vi "cDAQ_VI_Leo_Autotuning.vi"() -> ()   [LabVIEW 2022 SP3]
uses:
  <vilib>/addons/control/pid/autopid.llb/PID autotuning parameters.ctl
  <vilib>/Analysis/baseanly.llb/Mean (DBL).vi
  <vilib>/DAQmx/read.llb/DAQmx Read (Analog 1D Wfm NChan NSamp).vi
  STOP_GLOBAL.vi
  <vilib>/addons/control/pid/pid.llb/PID Lead-Lag (DBL).vi
  <vilib>/addons/control/pid/pid.llb/PID Gain Schedule (DBL).vi
  <vilib>/addons/control/pid/autopid.llb/PID Online Autotuning (Step Closed Loop).vi
  <vilib>/addons/control/pid/pid.llb/PID Advanced (DBL).vi
  <vilib>/addons/control/pid/pid.llb/PID (DBL).vi
  <vilib>/DAQmx/configure/timing.llb/DAQmx Timing (Sample Clock).vi
  <vilib>/DAQmx/miscellaneous.llb/DAQmx Fill In Error Info.vi
  <vilib>/Analysis/NI_AALBase.lvlib
  <vilib>/addons/control/pid/NI_PID_pid.lvlib
  <vilib>/ptbypt/NI_PtbyPt.lvlib
  <vilib>/addons/control/pid/NI_PID_autopid.lvlib
panel:
  in  "MV:":dbl(slide)=30.8641975308642 scale=1.0..5.067 scale format="%.1f"
  in  "autotuning parameters":T1={"type of controller"=0, "relay cycles"=3, "relay amplitude"=1.0, "control specifications"=2, "PV noise level"=0.1} {"PV noise level" format="%.2f"; "control specifications" items=["normal", "fast", "slow"]; "relay amplitude" format="%.2f"; "type of controller" items=["P", "PI", "PID"]}
  in  "PID gain schedule":T2(array[cluster])=[{"PID gains"={"Kc"=7.0, "Ti"=0.001, "Td"=0.0}, "max value"=0.0}] {"max value" format="%.2f"; "PID gains"."Td" format="%#.3g"; "PID gains"."Ti" format="%#.3g"; "PID gains"."Kc" format="%#.3g"}
  out "error out 4":errorcluster
  out "Setpoint profile":dbl
  out "Voltage Output":dynamicdata(graph)
  out "Second Pressure Transducer":cluster{dbl[], dbl[]}(graph)
  out "Second Pressure Transducer":dynamicdata(graph)
  out "Servo Voltage Output":cluster{dbl[], dbl[]}(graph)
  out "Elapsed Time (s)":dbl
  in  "Tab Control":T3(tab)
  in  "Channel Array":dbl[](array[numeric]) format="%_3g"
  out "error out 5":errorcluster
  in  "stop":bool
  out "Output":dbl(slide) scale=1.0..5.067
  out "elapsed time (s)":dbl format="%.3f"
  out "Waveform Chart 2":cluster{"setpoint":dbl, dbl}(graph) caption="Waveform Chart"
  out "Process Variable vs Setpoint":cluster{dbl[], dbl[]}[](graph)
  out "error out":errorcluster
  out "Steps on Needle 3":dbl[](array[numeric])
  in  "Error":dbl
  in  "Scaling Factor":dbl
  in  "x0":dbl
  out "element":dbl
  out "MVT Process variable":dbl
  out "MVT Setpoint":dbl
  out "Gain Index":i32
  in  "SP":dbl format="%.2f"
  out "PID gains out":T4={"proportional gain (Kc)"=1.0, "integral time (Ti, min)"=0.01, "derivative time (Td, min)"=0.0} {"derivative time (Td, min)" format="%.3f"; "integral time (Ti, min)" format="%.3f"; "proportional gain (Kc)" format="%.3f"}
  in  "Insert Gain":bool
  out "output":dbl format="%.2f"
  in  "Autotune":bool
  in  "Reinitialize":bool
  in  "Automatic":bool=TRUE
  in  "Replace Gain":bool
  in  "alpha":dbl=nan format="%.2f"
  out "tuned PID gains":T4={"proportional gain (Kc)"=1.0, "integral time (Ti, min)"=0.01, "derivative time (Td, min)"=0.0} {"derivative time (Td, min)" format="%.3f"; "integral time (Ti, min)" format="%.3f"; "proportional gain (Kc)" format="%.3f"}
  in  "EMERGENCY CLOSE":bool
  out "Steps on Servo":dbl[](array[numeric])
  out "Elapsed Time (s) 2":dbl caption="Elapsed Time (s)"
  out "HAS 3 SECONDS PASSED?":bool
  in  "PRESS TO START":bool
  out "All Channel Graph":cluster{dbl[], dbl[]}[](graph)
  out "Thrust":cluster{dbl[], dbl[]}(graph)
  out "Chamber Pressure":cluster{dbl[], dbl[]}(graph)
  out "Supply Pressure":cluster{dbl[], dbl[]}(graph)
  out "MassFlow":cluster{dbl[], dbl[]}(graph)
  out "Temperature":cluster{dbl[], dbl[]}(graph)
  out "error out 3":errorcluster caption="error out"
  out "error out 2":errorcluster
  in  "rate":dbl=1000.0 format="%0.2f"
  in  "number of samples":i32=100
  in  "File Format":string
  in  "File Name Out":string
  in  "Data Collection Folder":path
  out "Temperature":dynamicdata(graph)
  out "Numeric 2":i32
  out "Thrust lb":dynamicdata(graph)
  in  "Types of Testing":enum32{"Test Firing", "Cold Flow Rig"}(tab)
  out "Saving Data":bool
  out "Filename Out":path
  in  "Collect Data?":bool=TRUE caption="Enable"
  in  "Collect Data? 2":bool=TRUE caption="Enable"
  out "Saving Data":bool
  out "Filename Out":path
  out "Supply Pressure PSI":dynamicdata(graph)
  out "Mass Flow L/min":dynamicdata(graph)
  out "Chamber Pressure":dynamicdata(graph)
  # "Control Loop"
  # "DATA LOGGING INFORMATION"
  # "ANALOG VOLTAGE OUTPUT"
  # "RESULTS"
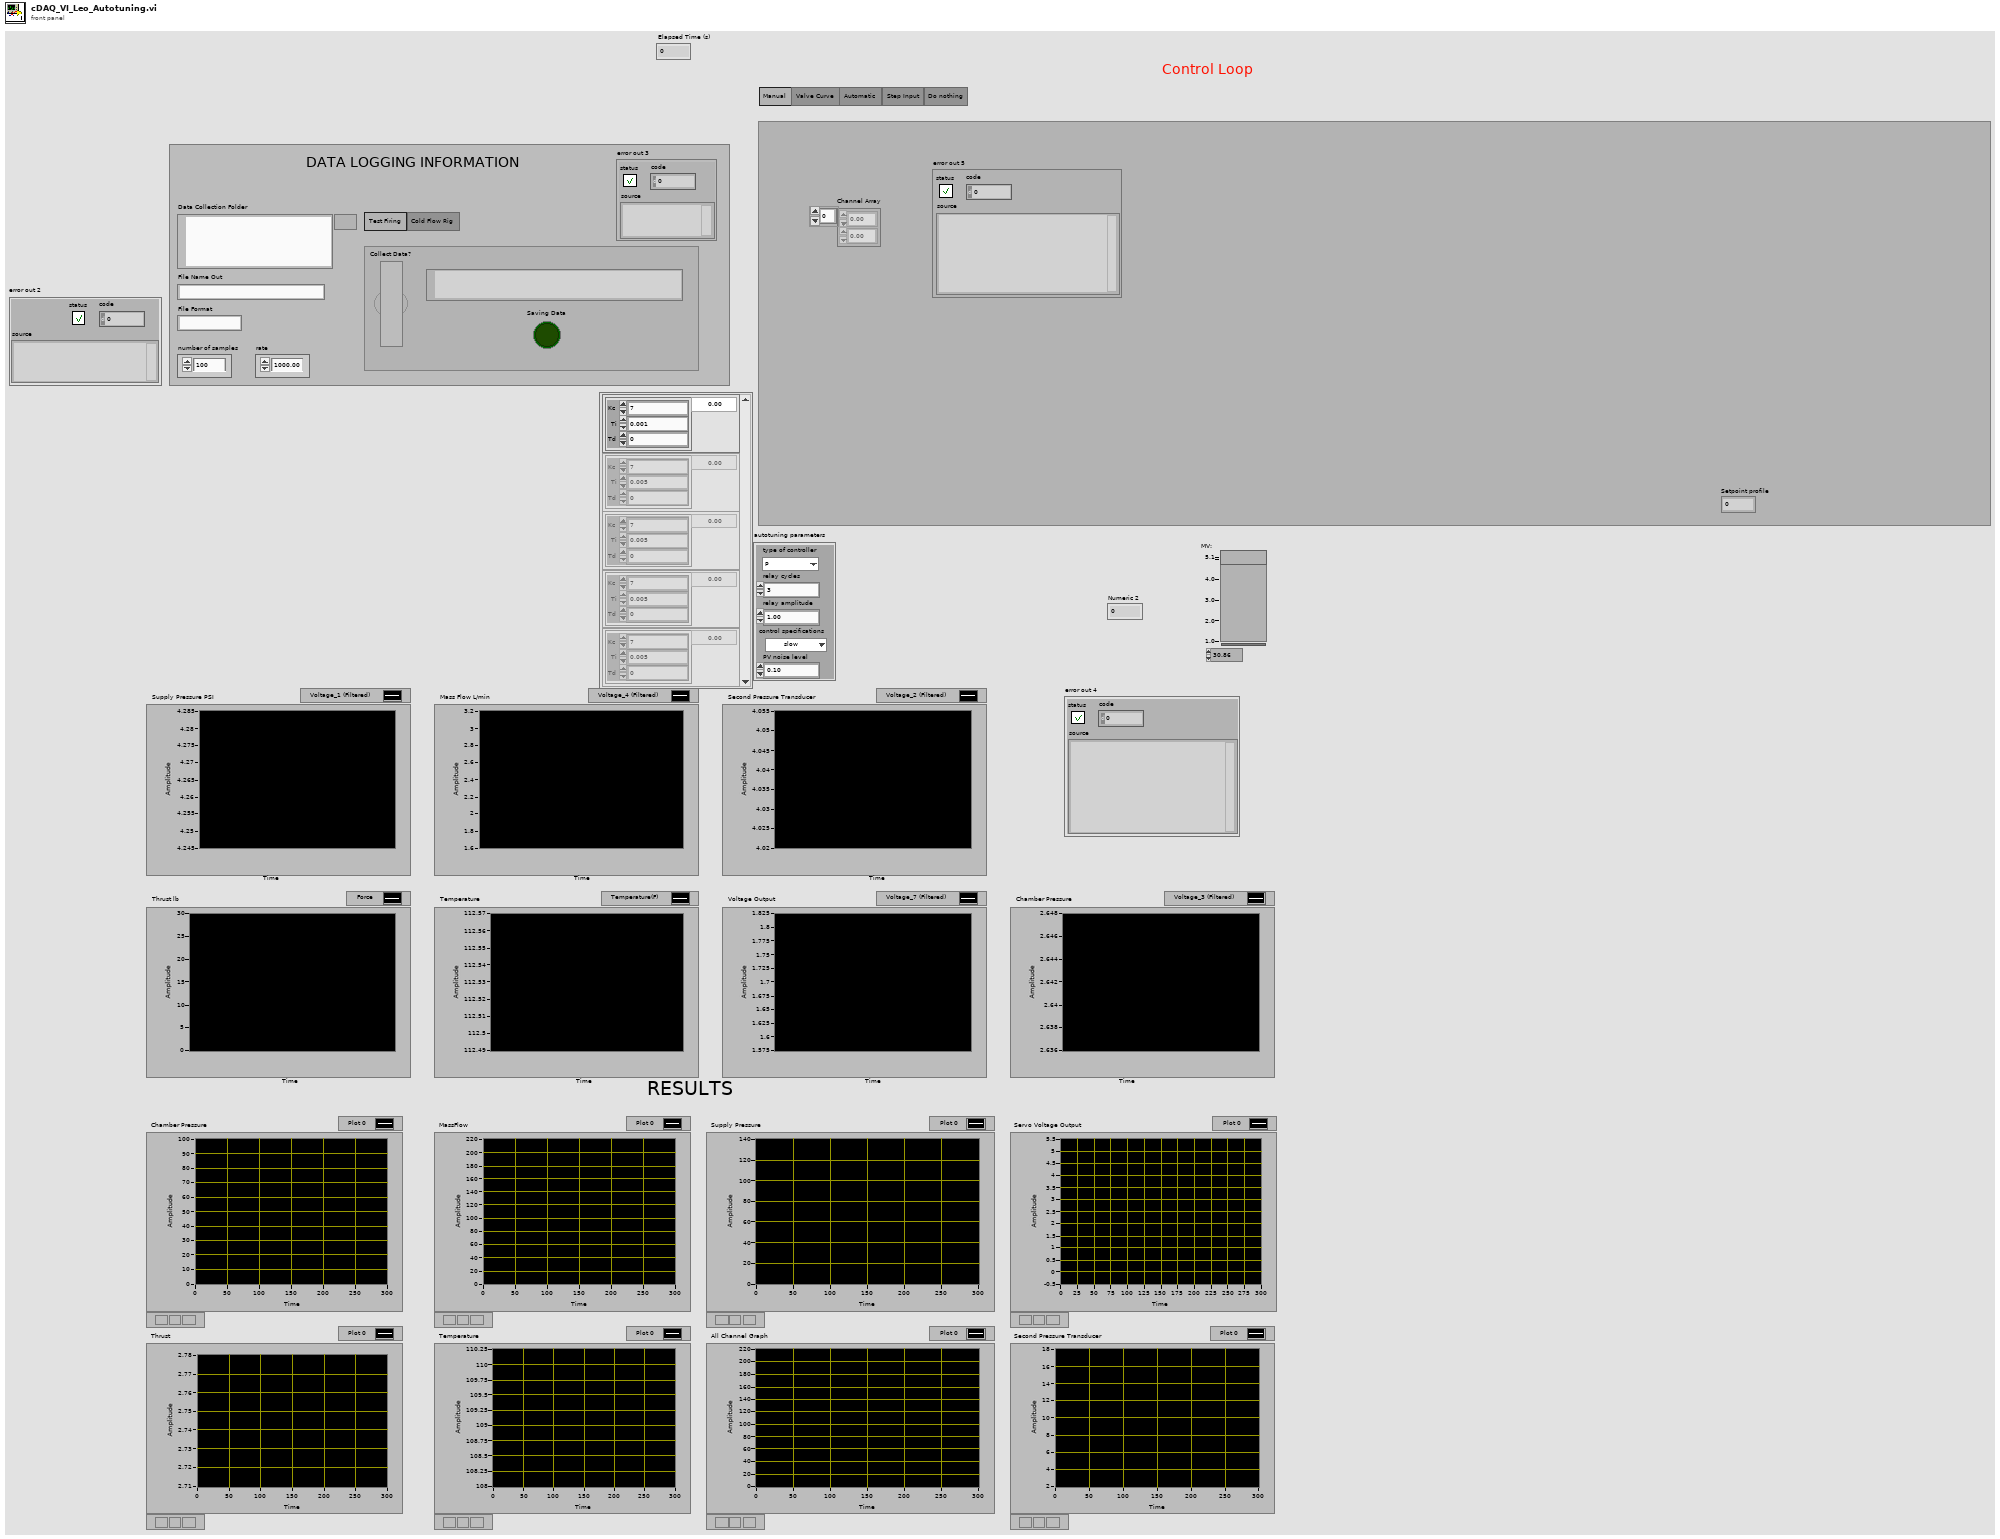
[diagram p1: front panel]
types:
  T1 = typedef "PID autotuning parameters.ctl" = cluster{"type of controller":u16, "relay cycles":i32, "relay amplitude":dbl, "control specifications":u16, "PV noise level":dbl}
  T2 = cluster{"PID gains":cluster{"Kc":dbl, "Ti":dbl, "Td":dbl}, "max value":dbl}[]
  T3 = enum32{"Manual", "Valve Curve", "Automatic", "Step Input", "Do nothing"}
  T4 = cluster{"proportional gain (Kc)":dbl, "integral time (Ti, min)":dbl, "derivative time (Td, min)":dbl}
  T5 = cluster{"tuned PID gains":cluster{"proportional gain (Kc)":dbl, "integral time (Ti, min)":dbl, "derivative time (Td, min)":dbl}, "SP":dbl}
  T6 = cluster{"PID gains":cluster{"Kc":dbl, "Ti":dbl, "Td":dbl}, "max value":dbl}
  T7 = cluster{"tuned PID gains":cluster{"proportional gain (Kc)":dbl, "integral time (Ti, min)":dbl, "derivative time (Td, min)":dbl}, "max value":dbl}
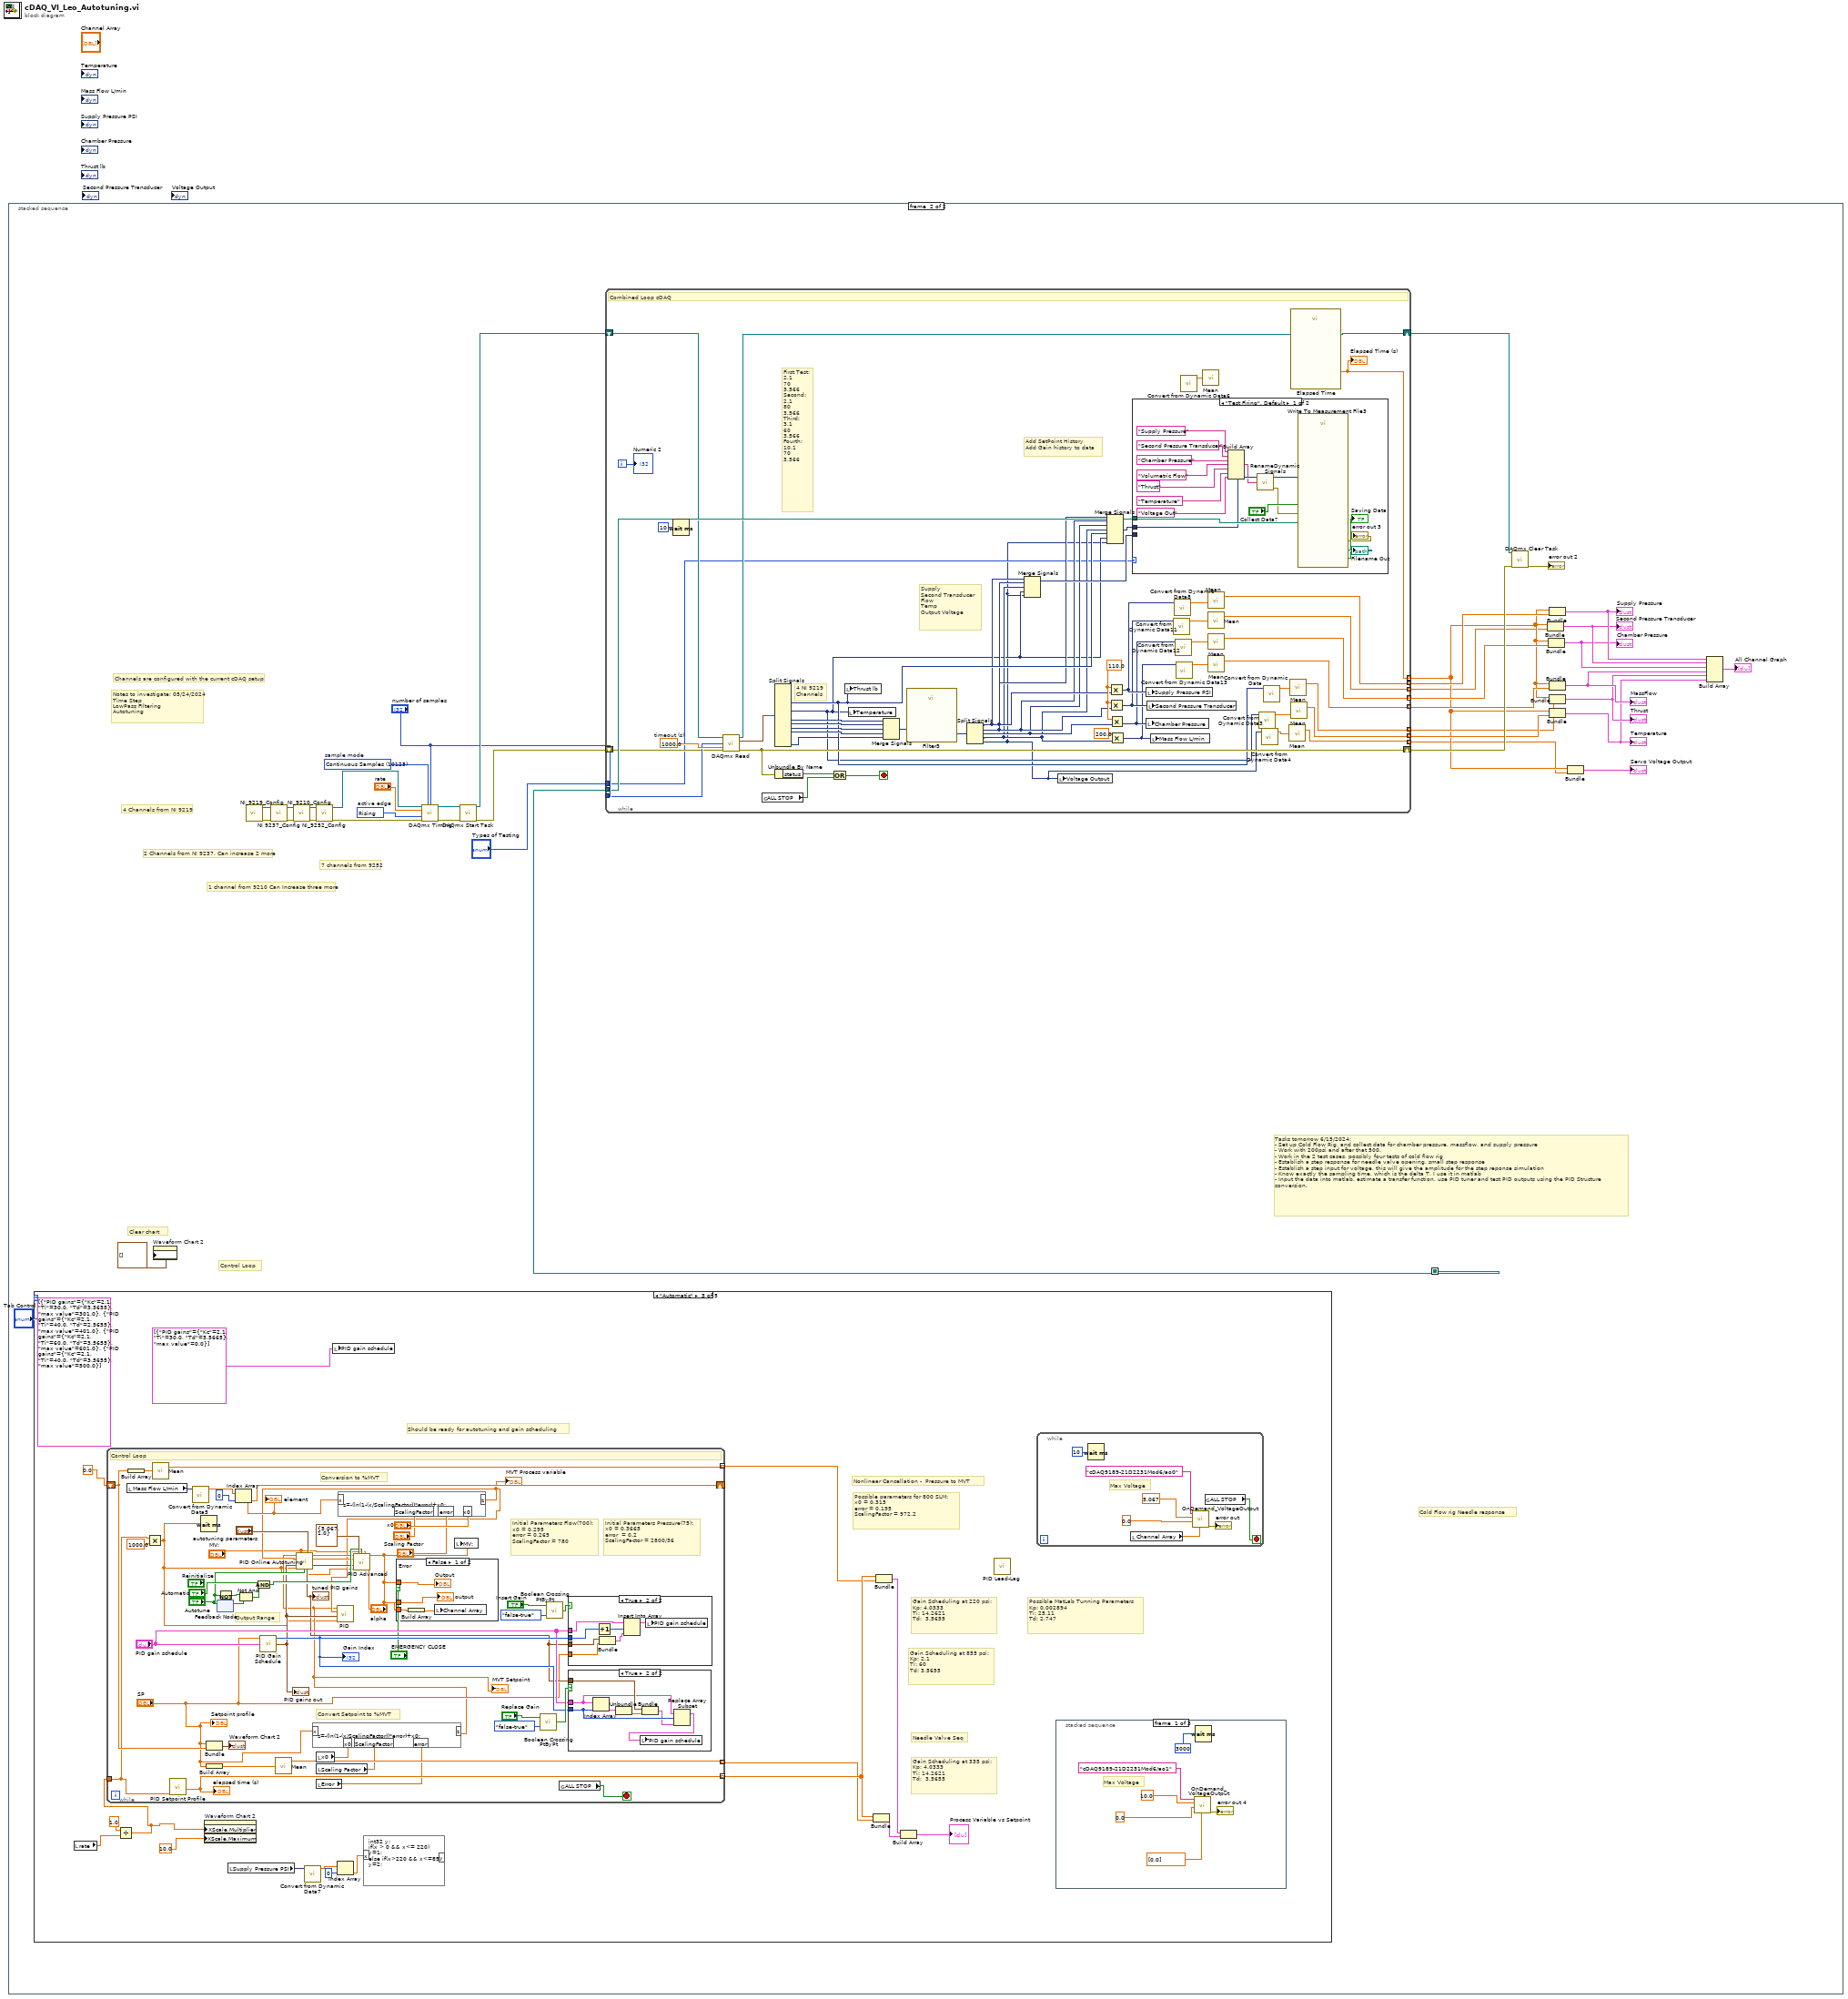
[diagram p0: block diagram]
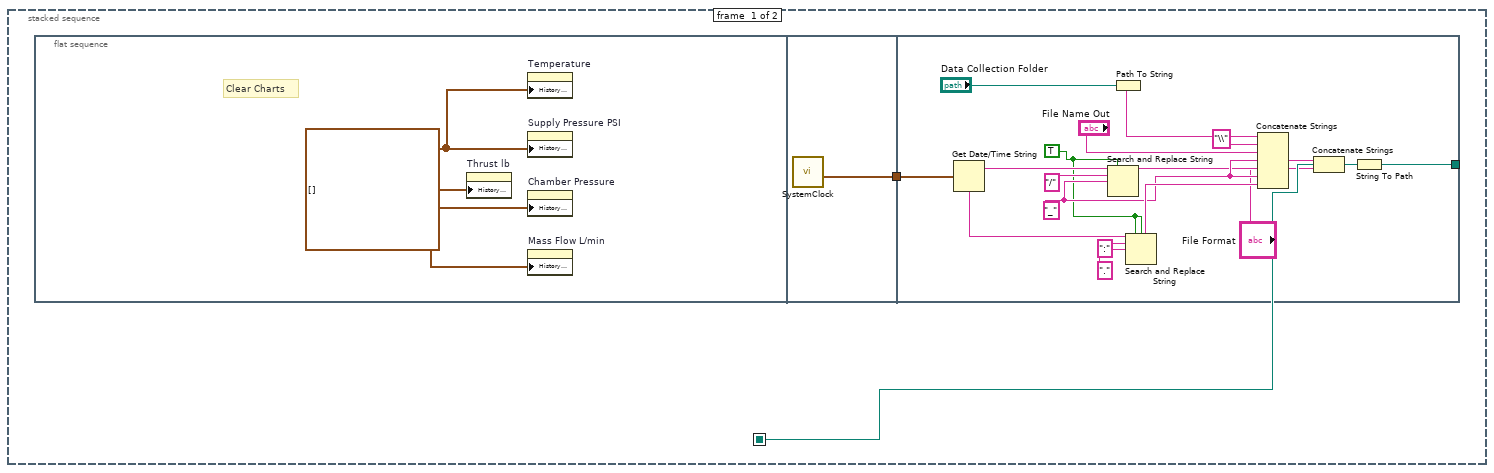
[diagram p2: hidden frame]
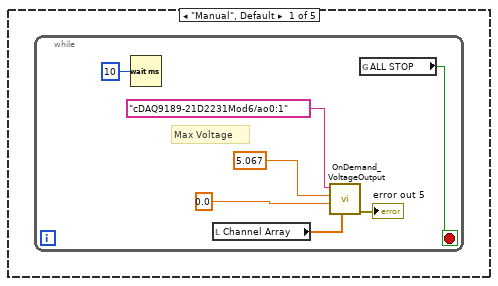
[diagram p3: hidden frame]
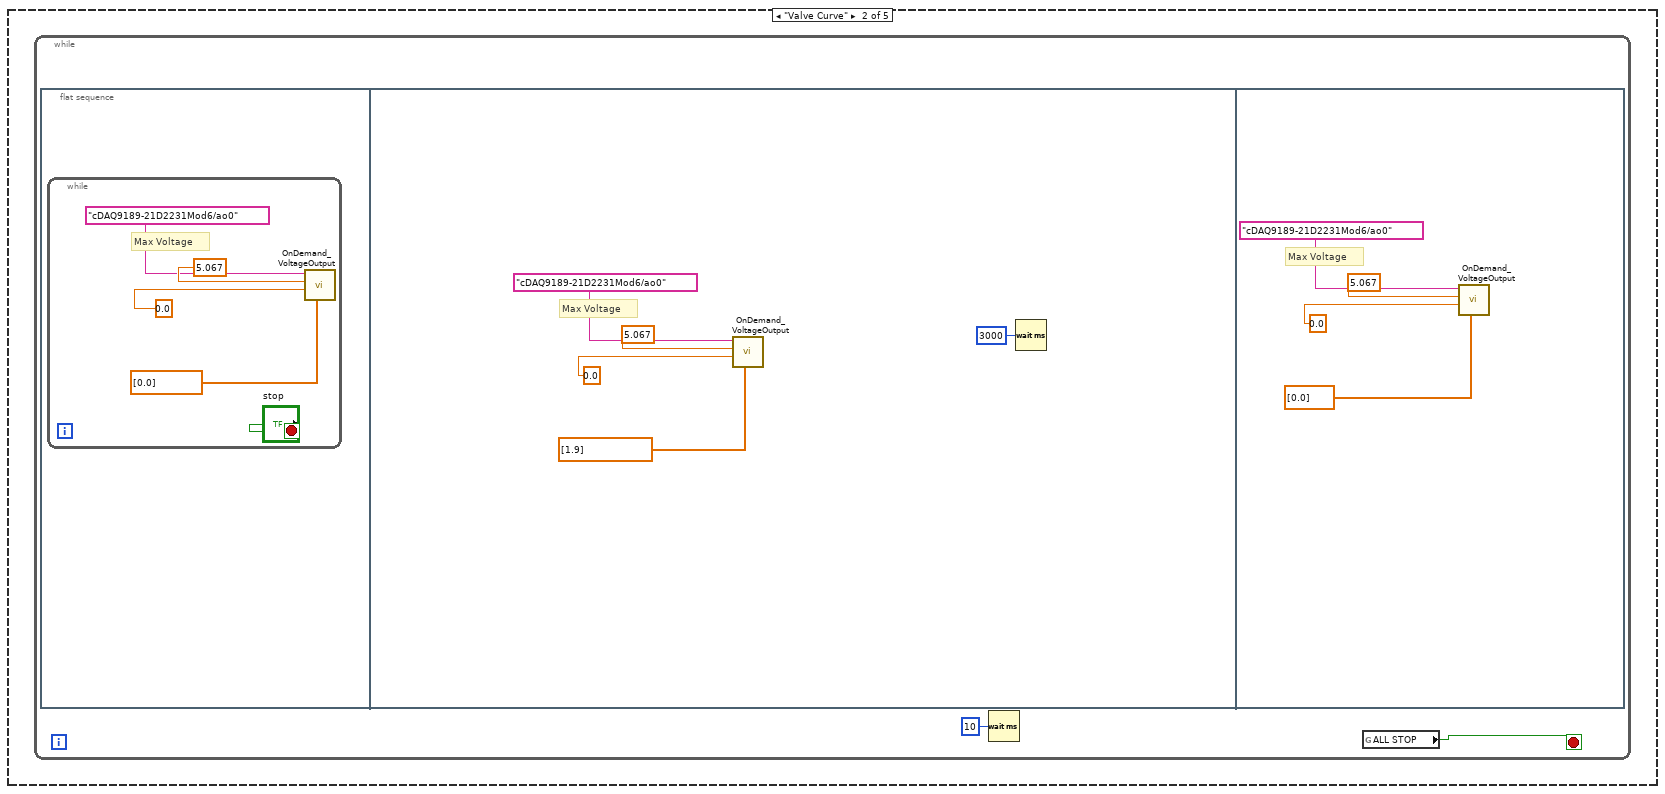
[diagram p4: hidden frame]
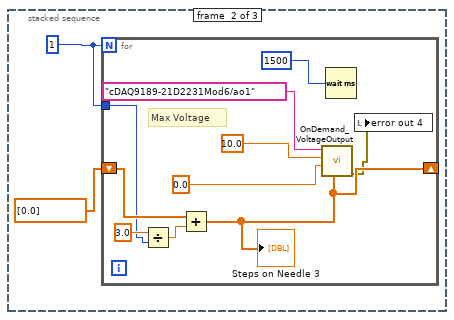
[diagram p5: hidden frame]
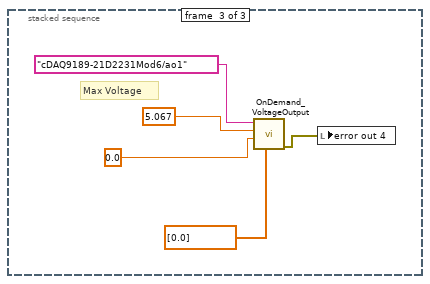
[diagram p6: hidden frame]
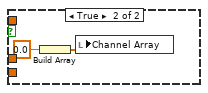
[diagram p7: hidden frame]
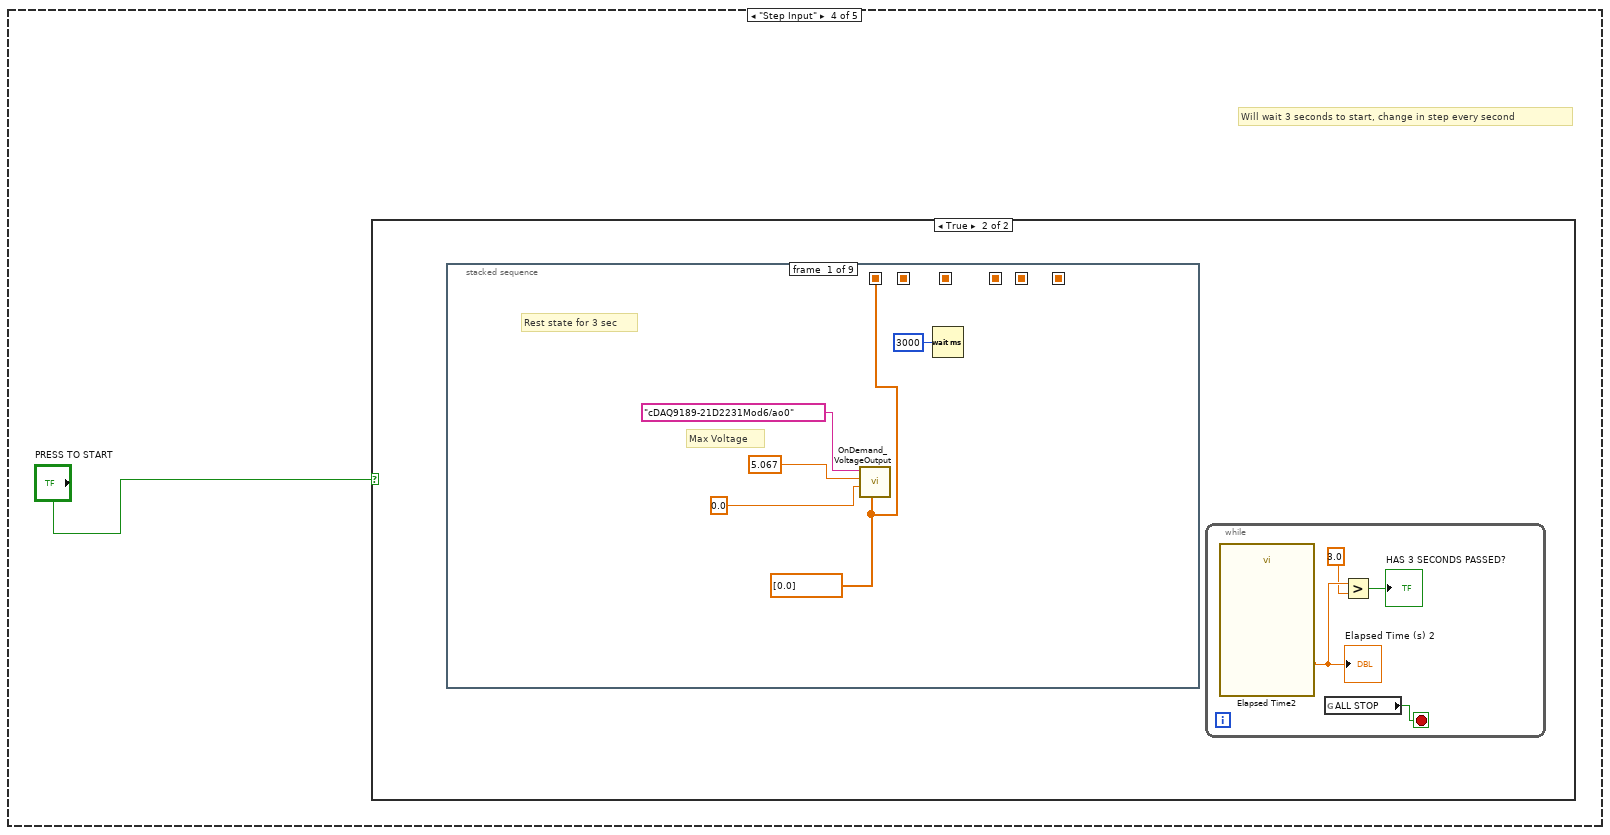
[diagram p10: hidden frame]
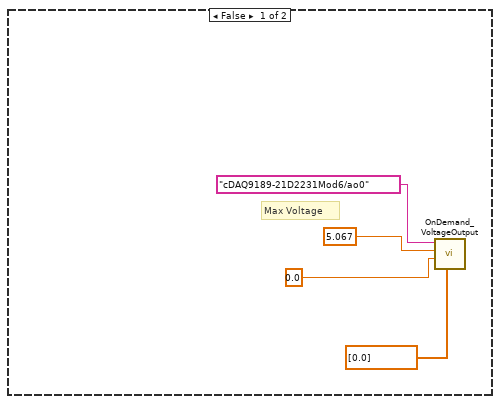
[diagram p11: hidden frame]
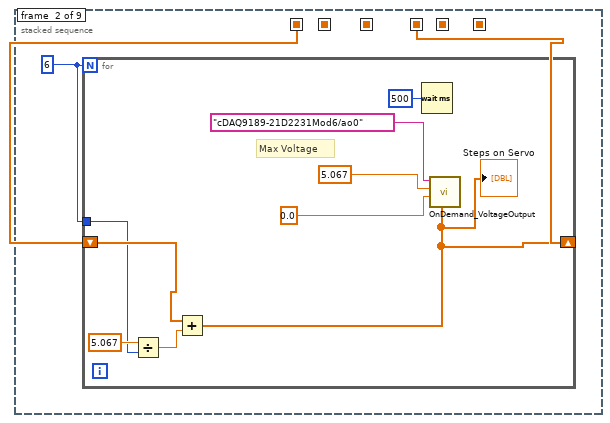
[diagram p12: hidden frame]
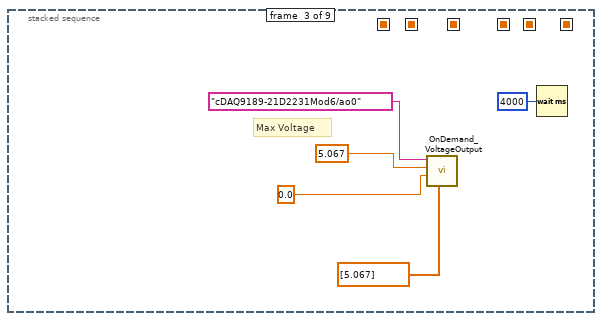
[diagram p13: hidden frame]
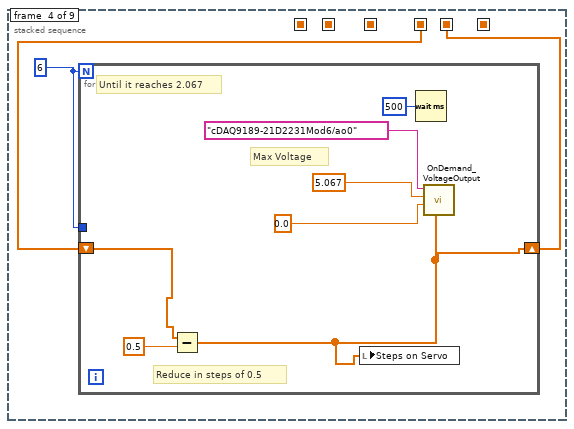
[diagram p14: hidden frame]
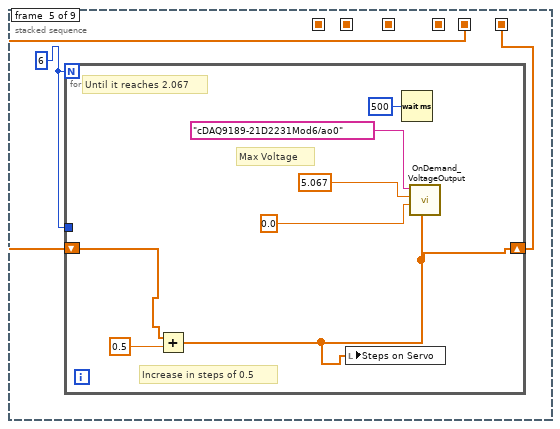
[diagram p15: hidden frame]
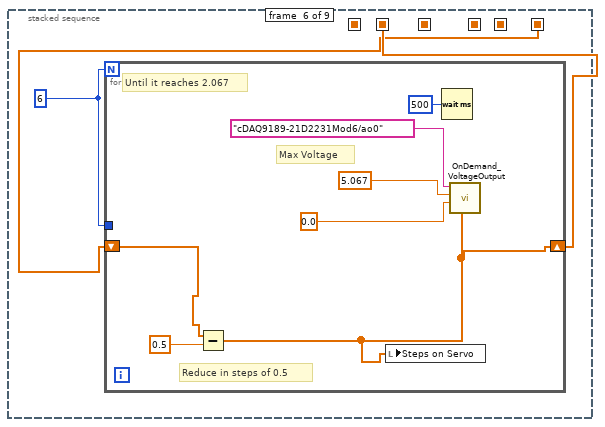
[diagram p16: hidden frame]
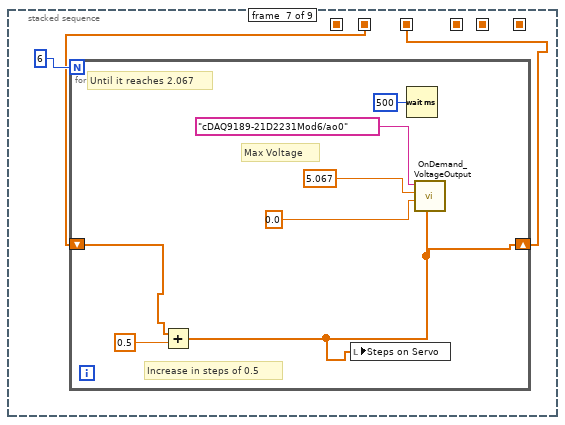
[diagram p17: hidden frame]
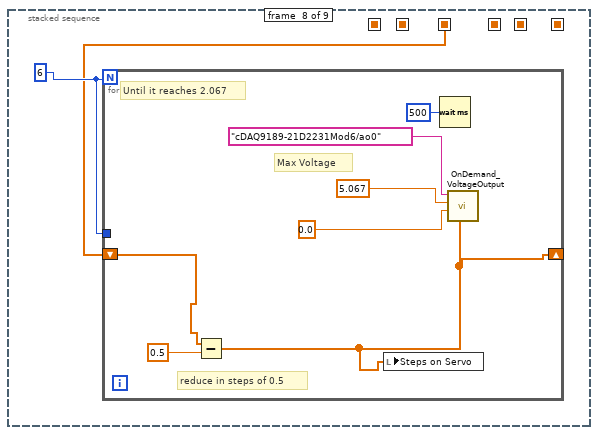
[diagram p18: hidden frame]
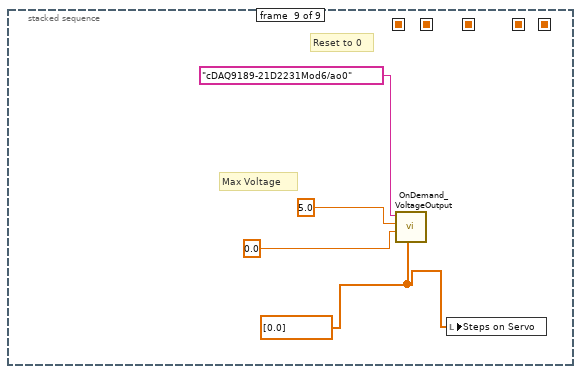
[diagram p19: hidden frame]
diagram:
  n1 = stacked-sequence {
    seq-local: [w1 _] -> [_ w60]
    frame #0 {
      n2 = flat-sequence {
        tunnel: [w4] -> w2
        tunnel: w2 -> [w11]
        tunnel: [w10] -> w1
        frame #0 {
          w3 = waveform(dbl)[] []
          # "Clear Charts"
          n3 = property on="Thrust lb" class="WFChart (strict)"("History Data"=w3) -> ()  [unwired: 2 in, 2 out]
          n4 = property on="Temperature" class="WFChart (strict)"("History Data"=w3) -> ()  [unwired: 2 in, 2 out]
          n5 = property on="Supply Pressure PSI" class="WFChart (strict)"("History Data"=w3) -> ()  [unwired: 2 in, 2 out]
          n6 = property on="Chamber Pressure" class="WFChart (strict)"("History Data"=w3) -> ()  [unwired: 2 in, 2 out]
          n7 = property on="Mass Flow L/min" class="WFChart (strict)"("History Data"=w3) -> ()  [unwired: 2 in, 2 out]
        }
        frame #1 {
          n8 = call "SystemClock.vi"() -> ("LabVIEW Time Stamp"=w4:timestamp)  [unwired: 9 in, 2 out]
        }
        frame #2 {
          w6 = TRUE ("replace all? (F)")
          w19 = "_" ("string")
          n9 = Get Date/Time String(seconds (now)=w11) -> (date string=w13:string, time string=w16:string)  [unwired: 2 in]
          n10 = Search and Replace String(replace all?=w6, input string=w13, search string="/", replace string=w19) -> (result string=w15:string)  [unwired: 4 in, 3 out]
          n11 = Path To String(path="Data Collection Folder") -> (string=w8:string)
          n12 = Search and Replace String(replace all?=w6, case sensitive?=w6, input string=w16, search string=":", replace string="." ("replace string (\"\")")) -> (result string=w20:string)  [unwired: 3 in, 3 out]
          n13 = Concatenate Strings(w8, "\\" ("string"), "File Name Out", w19, w15, w19, w20) -> (w21:string)
          n14 = Concatenate Strings(w21, "File Format") -> (w22:string)
          n15 = String To Path(string=w22) -> (path=w10:path)
        }
      }
    }
    frame #1 {
      w58 = 10123 items=["Finite Samples"=10178, "Continuous Samples"=10123, "Hardware Timed Single Point"=12522]  # sample mode
      w59 = 10280 items=["Rising"=10280, "Falling"=10171]  # active edge
      # "Cold Flow rig Needle response"
      # "Tasks tomorrow 6/15/2024:\n- Set up Cold Flow Rig, and collect data for chamber pressure, massflow, and supply pressure\n- Work with 200psi and after that 500.\n- Work in the 2 test cases, possibly four tests of cold flow rig\n- Establish a step response for needle valve opening, small step response\n- Establish a step input for voltage, this will give the amplitude for the step reponse simulation\n- Know exactly the sampling time, which is the delta T, I use it in matlab\n- Input the data into matlab, estimate a transfer function, use PID tuner and test PID outputs using the PID Structure\nconversion."
      # "Control Loop"
      # "Clear chart"
      # "Notes to investigate: 05/24/2024\nTime Step\nLowPass FIltering\nAutotuning"
      # "Channels are configured with the current cDAQ setup"
      # "7 channels from 9252"
      # "1 channel from 9210 Can Increase three more"
      # "2 Channels from NI 9237, Can increase 2 more"
      # "4 Channels from NI 9219"
      n16 = case shown="\"Automatic\"" "Tab Control" {
        frame "Manual", Default {
          n17 = while {
            stop <- w68 stop-if-true
            # "Max Voltage"
            n18 = Wait (ms)(milliseconds to wait=u32 10) -> ()  [unwired: 1 out]
            n19 = local read "Channel Array"() -> (w64:dbl[])
            n20 = call "OnDemand_VoltageOutput.vi"("Channel Array"=w64, "minimum voltage"=0.0, "maximum voltage"=5.067, "physical channels"="cDAQ9189-21D2231Mod6/ao0:1") -> ("error out"=→"error out 5":errorcluster)  [unwired: 7 in]
            n21 = global read "STOP_GLOBAL.vi" "ALL STOP"() -> (w68:bool)
          }
        }
        frame "Valve Curve" {
          n22 = while {
            stop <- w69 stop-if-true
            n23 = flat-sequence {
              frame #0 {
                n24 = while {
                  stop <- "stop" stop-if-true
                  # "Max Voltage"
                  n25 = call "OnDemand_VoltageOutput.vi"("Channel Array"=dbl[] [0.0], "minimum voltage"=0.0, "maximum voltage"=5.067, "physical channels"="cDAQ9189-21D2231Mod6/ao0") -> ()  [unwired: 7 in, 1 out]
                }
              }
              frame #1 {
                # "Max Voltage"
                n26 = call "OnDemand_VoltageOutput.vi"("Channel Array"=dbl[] [1.9], "minimum voltage"=0.0, "maximum voltage"=5.067, "physical channels"="cDAQ9189-21D2231Mod6/ao0") -> ()  [unwired: 7 in, 1 out]
                n27 = Wait (ms)(milliseconds to wait=u32 3000) -> ()  [unwired: 1 out]
              }
              frame #2 {
                # "Max Voltage"
                n28 = call "OnDemand_VoltageOutput.vi"("Channel Array"=dbl[] [0.0], "minimum voltage"=0.0, "maximum voltage"=5.067, "physical channels"="cDAQ9189-21D2231Mod6/ao0") -> ()  [unwired: 7 in, 1 out]
              }
            }
            n29 = Wait (ms)(milliseconds to wait=u32 10) -> ()  [unwired: 1 out]
            n30 = global read "STOP_GLOBAL.vi" "ALL STOP"() -> (w69:bool)
          }
        }
        frame "Automatic" {
          (unwired) T2 [{"PID gains"={"Kc"=2.1, "Ti"=30.0, "Td"=3.5655}, "max value"=301.0}, {"PID gains"={"Kc"=2.1, "Ti"=40.0, "Td"=2.5655}, "max value"=401.0}, {"PID gains"={"Kc"=2.1, "Ti"=60.0, "Td"=3.5655}, "max value"=601.0}, {"PID gains"={"Kc"=2.1, "Ti"=40.0, "Td"=3.5655}, "max value"=500.0}] ("PID gain schedule 2")
          # "Should be ready for autotuning and gain scheduling"
          # "Possible parameters for 800 SLM:\nx0 = 0.315\nerror = 0.195\nScalingFactor = 972.2"
          # "Nonlinear Cancellation -  Pressure to MVT"
          # "Possible MatLab Tunning Parameters\nKp: 0.002894\nTi: 25.11\nTd: 2.747"
          # "Gain Scheduling at 335 psi:\nKp: 4.0333\nTi: 14.2621\nTd:  3.5655"
          # "Gain Scheduling at 855 psi:\nKp: 2.1\nTi: 60\nTd: 3.5655"
          # "Gain Scheduling at 220 psi:\nKp: 4.0333\nTi: 14.2621\nTd:  3.5655"
          # "Needle Valve Seq"
          n31 = local read "rate"() -> (w85:dbl)
          n32 = Divide(x=1.0, y=w85) -> (x/y=w88:dbl)
          n33 = while {
            shift-right: [w138] -> _
            shift-left: 0.0 -> [w176]
            tunnel: w88 -> [w139]
            tunnel: [w177] -> w97 mode=indexing
            tunnel: [w175] -> w95 mode=indexing
            tunnel: [w173] -> w96 mode=indexing
            stop <- w179 stop-if-true
            # "Initial Parameters Pressure(75):\nx0 = 0.3665\nerror  = 0.2\nScalingFactor = 2800/36"
            # "Initial Parameters Flow(700):\nx0 = 0.295\nerror = 0.265\nScalingFactor = 780"
            # "Convert Setpoint to %MVT"
            # "Conversion to %MVT"
            # "Output Range"
            # "Control Loop"
            n34 = local read "Mass Flow L/min"() -> (w163:dynamicdata)
            n35 = Build Array(w176) -> (w174:dbl[])
            n36 = Multiply(x=w139, y=1000.0) -> (x*y=w131:dbl)
            n37 = call-poly <vilib>:"Mean.vi"("X"=w174) -> ("mean"=w175:dbl)  [unwired: 1 out]
            n38 = call <vilib>:"PID Setpoint Profile.vi"("dt (s)"=w139) -> ("elapsed time (s)"=w177:dbl)  [unwired: 5 in, 3 out]
            "elapsed time (s)" <- w177
            n39 = call "Convert from Dynamic Data5"("Dynamic Data Type"=w163) -> ("Array"=w164:dbl[])  [unwired: 3 in]
            n40 = Wait (ms)(milliseconds to wait=w131) -> ()  [unwired: 1 out]
            n41 = Bundle("SP"="SP", w176) -> (→"Waveform Chart 2":cluster{"SP":dbl, dbl})  [unwired: 1 in]
            n42 = Build Array("SP") -> (w170:dbl[])
            n43 = feedback #1() -> (w158:bool)  [unwired: 1 in]
            n44 = feedback-in #1("Autotune") -> ()
            n45 = Not(x="Autotune") -> (.not. x?=w157:bool)
            n46 = Index Array(array=w164, index=0) -> (element=w138:dbl)
            "element" <- w138
            n47 = Not And(1:w158, 2:w157) -> (0:w156:bool)
            n48 = And(x="Automatic", y=w156) -> (x .and. y?=w152:bool)
            n49 = call-poly <vilib>:"PID Gain Schedule.vi"("PID gain schedule"="PID gain schedule", "gain scheduling value"="SP") -> ("PID gains out"=w142:T4, "index out"=w144:i32)  [unwired: 2 in]
            "Gain Index" <- w144
            "PID gains out" <- w142
            n50 = call-poly <vilib>:"Mean.vi"("X"=w170) -> ("mean"=w173:dbl)  [unwired: 1 out]
            n51 = local read "x0"() -> (w169:dbl)
            n52 = local read "Scaling Factor"() -> (w159:dbl)
            n53 = local read "Error"() -> (w168:dbl)
            n54 = formula code="z=-(ln(1-(x/ScalingFactor))*error)+x0;"("x"="SP", "x0"=w169, "ScalingFactor"=w159, "error"=w168) -> ("z"=w135:dbl)
            "MVT Setpoint" <- w135
            n55 = formula code="z=-(ln(1-(x/ScalingFactor))*error)+x0;"("x"=w138, "x0"="x0", "ScalingFactor"="Scaling Factor", "error"="Error") -> ("z"=w137:dbl)
            "MVT Process variable" <- w137
            n56 = call-poly <vilib>:"PID Online Autotuning.vi"("setpoint"=w135, "manipulated variable"="MV:", "autotuning parameters"="autotuning parameters", "process variable"=w137, "PID gains in"=w142, "dt (s)"=w131, "autotune? (F)"="Autotune") -> ("setpoint out"=w151:dbl, "process variable out"=w150:dbl, "PID gains out"=w149:T4, "tuned PID gains"=w140:T4)  [unwired: 4 in, 1 out]
            "tuned PID gains" <- w140
            n57 = call-poly <vilib>:"PID.vi"("dt (s)"=w131, "PID gains"=w142, "process variable"=w137, "setpoint"=w135) -> ()  [unwired: 6 in, 2 out]
            n58 = call-poly <vilib>:"PID Advanced.vi"("setpoint"=w151, "output range"=cluster{"output high":dbl, "output low":dbl} {"output high"=5.067, "output low"=1.0}, "auto? (T)"=w152, "manual control"="MV:", "process variable"=w150, "alpha"="alpha", "PID gains"=w149, "dt (s)"=w131) -> ("output"=w132:dbl)  [unwired: 6 in, 1 out]
            n59 = case shown="False" "EMERGENCY CLOSE" {
              tunnel: w132 -> [w183 _]
              tunnel: w132 -> [w182 _]
              tunnel: w132 -> [w180 _]
              frame False {
                n60 = Build Array(w180) -> (w181:dbl[])
                n61 = local write "Channel Array"(w181) -> ()
                "Output" <- w183
                "output" <- w182
              }
              frame True {
                n62 = Build Array(0.0 ("element")) -> (w185:dbl[])
                n63 = local write "Channel Array"(w185) -> ()
              }
            }
            n64 = local write "MV:"(w132) -> ()
            n65 = call <vilib>:"Boolean Crossing PtByPt.vi"("direction"=enum16{"either", "false-true", "true-false"}."false-true", "input"="Replace Gain") -> ("crossing"=w145:bool)  [unwired: 1 in]
            n66 = call <vilib>:"Boolean Crossing PtByPt.vi"("direction"=enum16{"either", "false-true", "true-false"}."false-true", "input"="Insert Gain") -> ("crossing"=w161:bool)  [unwired: 1 in]
            n67 = global read "STOP_GLOBAL.vi" "ALL STOP"() -> (w179:bool)
            n68 = case shown="True" w161 {
              tunnel: w144 -> [_ w199]
              tunnel: "PID gain schedule" -> [_ w197]
              tunnel: "SP" -> [_ w196]
              tunnel: w140 -> [_ w194]
              frame False {
              }
              frame True {
                n69 = Increment(x=w199) -> (x+1=w198:i32)
                n70 = Bundle("tuned PID gains"=w194, "SP"=w196) -> (w193:T5)  [unwired: 1 in]
                n71 = Insert Into Array(array=w197, index=w198, new element=w193) -> (w195:T2)
                n72 = local write "PID gain schedule"(w195) -> ()
              }
            }
            n73 = case shown="True" w145 {
              tunnel: w144 -> [_ w189]
              tunnel: "PID gain schedule" -> [_ w187]
              tunnel: w140 -> [_ w190]
              frame False {
              }
              frame True {
                n74 = Index Array(array=w187, index=w189) -> (element=w192:T6)
                n75 = Unbundle(w192) -> ("max value"=w191:dbl)  [unwired: 1 out]
                n76 = Bundle("tuned PID gains"=w190, "max value"=w191) -> (w188:T7)  [unwired: 1 in]
                n77 = Replace Array Subset(array=w187, new element=w188, index=w189) -> (w186:T2)
                n78 = local write "PID gain schedule"(w186) -> ()
              }
            }
            "Setpoint profile" <- "SP"
          }
          n79 = property on="Waveform Chart 2" class="WFChart (strict)"("XScale.Multiplier"=w88, "XScale.Maximum"=10.0 ("X Scale.Range:Maximum")) -> ()  [unwired: 2 in, 2 out]
          n80 = local read "Supply Pressure PSI"() -> (w92:dynamicdata)
          n81 = call "Convert from Dynamic Data7"("Dynamic Data Type"=w92) -> ("Array"=w91:dbl[])  [unwired: 3 in]
          n82 = local write "PID gain schedule"(T2 [{"PID gains"={"Kc"=2.1, "Ti"=30.0, "Td"=3.5665}, "max value"=0.0}] ("PID gain schedule 2")) -> ()
          n83 = Index Array(array=w91, index=0) -> (element=w89:dbl)
          n84 = formula code="int32 y;\nif(x > 0 && x<= 220)\ny=1;\nelse if(x>220 && x<=855)\ny=2;"("x"=w89) -> ()  [unwired: 1 out]
          n85 = Bundle(w97, w96) -> (w98:cluster{dbl[], dbl[]})  [unwired: 1 in]
          n86 = Bundle(w97, w95) -> (w93:cluster{dbl[], dbl[]})  [unwired: 1 in]
          n87 = Build Array(w93, w98) -> (→"Process Variable vs Setpoint":cluster{dbl[], dbl[]}[])
          n88 = call-poly <vilib>:"PID Lead-Lag.vi"() -> ()  [unwired: 8 in, 2 out]
          n89 = while {
            stop <- w130 stop-if-true
            # "Max Voltage"
            n90 = Wait (ms)(milliseconds to wait=u32 10) -> ()  [unwired: 1 out]
            n91 = local read "Channel Array"() -> (w126:dbl[])
            n92 = call "OnDemand_VoltageOutput.vi"("Channel Array"=w126, "minimum voltage"=0.0, "maximum voltage"=5.067, "physical channels"="cDAQ9189-21D2231Mod6/ao0") -> ("error out"=→"error out":errorcluster)  [unwired: 7 in]
            n93 = global read "STOP_GLOBAL.vi" "ALL STOP"() -> (w130:bool)
          }
          n94 = stacked-sequence {
            frame #0 {
              # "Max Voltage"
              n95 = call "OnDemand_VoltageOutput.vi"("Channel Array"=dbl[] [0.0], "minimum voltage"=0.0, "maximum voltage"=10.0, "physical channels"="cDAQ9189-21D2231Mod6/ao1") -> ("error out"=→"error out 4":errorcluster)  [unwired: 7 in]
              n96 = Wait (ms)(milliseconds to wait=u32 3000) -> ()  [unwired: 1 out]
            }
            frame #1 {
              w107 = 1
              n97 = for {
                N: w107 -> [_]
                shift-right: [w110] -> _
                shift-left: dbl[] [0.0] -> [w114]
                tunnel: w107 -> [w112]
                # "Max Voltage"
                n98 = Divide(x=3.0, y=w112) -> (x/y=w111:dbl)
                n99 = Add(x=w114, y=w111) -> (x+y=w110:dbl[])
                "Steps on Needle 3" <- w110
                n100 = call "OnDemand_VoltageOutput.vi"("Channel Array"=w110, "minimum voltage"=0.0, "maximum voltage"=10.0, "physical channels"="cDAQ9189-21D2231Mod6/ao1") -> ("error out"=w109:errorcluster)  [unwired: 7 in]
                n101 = Wait (ms)(milliseconds to wait=u32 1500) -> ()  [unwired: 1 out]
                n102 = local write "error out 4"(w109) -> ()
              }
            }
            frame #2 {
              # "Max Voltage"
              n103 = call "OnDemand_VoltageOutput.vi"("Channel Array"=dbl[] [0.0], "minimum voltage"=0.0, "maximum voltage"=5.067, "physical channels"="cDAQ9189-21D2231Mod6/ao1") -> ("error out"=w119:errorcluster)  [unwired: 7 in]
              n104 = local write "error out 4"(w119) -> ()
            }
          }
        }
        frame "Step Input" {
          # "Will wait 3 seconds to start, change in step every second"
          n105 = case shown="True" "PRESS TO START" {
            frame False {
              # "Max Voltage"
              n106 = call "OnDemand_VoltageOutput.vi"("Channel Array"=dbl[] [0.0], "minimum voltage"=0.0, "maximum voltage"=5.067, "physical channels"="cDAQ9189-21D2231Mod6/ao0") -> ()  [unwired: 7 in, 1 out]
            }
            frame True {
              n107 = stacked-sequence {
                seq-local: [_ _ _ _ _ w252 _ _ _] -> [_ _ _ _ _ _ w262 _ _]
                seq-local: [_ _ _ _ _ _ w261 _ _] -> [_ _ _ _ _ _ _ w271 _]
                seq-local: [w209 _ _ _ _ _ _ _ _] -> [_ w215 _ _ _ _ _ _ _]
                seq-local: [_ w214 _ _ _ _ _ _ _] -> [_ _ _ w232 _ _ _ _ _]
                seq-local: [_ _ _ w231 _ _ _ _ _] -> [_ _ _ _ w242 _ _ _ _]
                seq-local: [_ _ _ _ w241 _ _ _ _] -> [_ _ _ _ _ w251 _ _ _]
                frame #0 {
                  w209 = dbl[] [0.0]
                  # "Rest state for 3 sec"
                  # "Max Voltage"
                  n108 = call "OnDemand_VoltageOutput.vi"("Channel Array"=w209, "minimum voltage"=0.0, "maximum voltage"=5.067, "physical channels"="cDAQ9189-21D2231Mod6/ao0") -> ()  [unwired: 7 in, 1 out]
                  n109 = Wait (ms)(milliseconds to wait=u32 3000) -> ()  [unwired: 1 out]
                }
                frame #1 {
                  w216 = 6
                  n110 = for {
                    N: w216 -> [_]
                    shift-right: [w217] -> w214
                    shift-left: w215 -> [w224]
                    tunnel: w216 -> [w218]
                    # "Max Voltage"
                    n111 = Divide(x=5.067, y=w218) -> (x/y=w220:dbl)
                    n112 = Add(x=w224, y=w220) -> (x+y=w217:dbl[])
                    "Steps on Servo" <- w217
                    n113 = Wait (ms)(milliseconds to wait=u32 500) -> ()  [unwired: 1 out]
                    n114 = call "OnDemand_VoltageOutput.vi"("Channel Array"=w217, "minimum voltage"=0.0, "maximum voltage"=5.067, "physical channels"="cDAQ9189-21D2231Mod6/ao0") -> ()  [unwired: 7 in, 1 out]
                  }
                }
                frame #2 {
                  # "Max Voltage"
                  n115 = call "OnDemand_VoltageOutput.vi"("Channel Array"=dbl[] [5.067], "minimum voltage"=0.0, "maximum voltage"=5.067, "physical channels"="cDAQ9189-21D2231Mod6/ao0") -> ()  [unwired: 7 in, 1 out]
                  n116 = Wait (ms)(milliseconds to wait=u32 4000) -> ()  [unwired: 1 out]
                }
                frame #3 {
                  w233 = 6
                  n117 = for {
                    N: w233 -> [_]
                    shift-right: [w234] -> w231
                    shift-left: w232 -> [w240]
                    tunnel: w233 -> [_]
                    # "Max Voltage"
                    # "Until it reaches 2.067"
                    # "Reduce in steps of 0.5"
                    n118 = Subtract(x=w240, y=0.5) -> (x-y=w234:dbl[])
                    n119 = local write "Steps on Servo"(w234) -> ()
                    n120 = Wait (ms)(milliseconds to wait=u32 500) -> ()  [unwired: 1 out]
                    n121 = call "OnDemand_VoltageOutput.vi"("Channel Array"=w234, "minimum voltage"=0.0, "maximum voltage"=5.067, "physical channels"="cDAQ9189-21D2231Mod6/ao0") -> ()  [unwired: 7 in, 1 out]
                  }
                }
                frame #4 {
                  w243 = 6
                  n122 = for {
                    N: w243 -> [_]
                    shift-right: [w244] -> w241
                    shift-left: w242 -> [w250]
                    tunnel: w243 -> [_]
                    # "Max Voltage"
                    # "Until it reaches 2.067"
                    # "Increase in steps of 0.5"
                    n123 = Add(x=w250, y=0.5) -> (x+y=w244:dbl[])
                    n124 = local write "Steps on Servo"(w244) -> ()
                    n125 = Wait (ms)(milliseconds to wait=u32 500) -> ()  [unwired: 1 out]
                    n126 = call "OnDemand_VoltageOutput.vi"("Channel Array"=w244, "minimum voltage"=0.0, "maximum voltage"=5.067, "physical channels"="cDAQ9189-21D2231Mod6/ao0") -> ()  [unwired: 7 in, 1 out]
                  }
                }
                frame #5 {
                  w253 = 6
                  n127 = for {
                    N: w253 -> [_]
                    shift-right: [w254] -> w252
                    shift-left: w251 -> [w260]
                    tunnel: w253 -> [_]
                    # "Max Voltage"
                    # "Until it reaches 2.067"
                    # "Reduce in steps of 0.5"
                    n128 = Subtract(x=w260, y=0.5) -> (x-y=w254:dbl[])
                    n129 = local write "Steps on Servo"(w254) -> ()
                    n130 = Wait (ms)(milliseconds to wait=u32 500) -> ()  [unwired: 1 out]
                    n131 = call "OnDemand_VoltageOutput.vi"("Channel Array"=w254, "minimum voltage"=0.0, "maximum voltage"=5.067, "physical channels"="cDAQ9189-21D2231Mod6/ao0") -> ()  [unwired: 7 in, 1 out]
                  }
                }
                frame #6 {
                  n132 = for {
                    N: 6 -> [_]
                    shift-right: [w264] -> w261
                    shift-left: w262 -> [w270]
                    # "Max Voltage"
                    # "Until it reaches 2.067"
                    # "Increase in steps of 0.5"
                    n133 = Add(x=w270, y=0.5) -> (x+y=w264:dbl[])
                    n134 = local write "Steps on Servo"(w264) -> ()
                    n135 = Wait (ms)(milliseconds to wait=u32 500) -> ()  [unwired: 1 out]
                    n136 = call "OnDemand_VoltageOutput.vi"("Channel Array"=w264, "minimum voltage"=0.0, "maximum voltage"=5.067, "physical channels"="cDAQ9189-21D2231Mod6/ao0") -> ()  [unwired: 7 in, 1 out]
                  }
                }
                frame #7 {
                  w272 = 6
                  n137 = for {
                    N: w272 -> [_]
                    shift-right: [w273] -> _
                    shift-left: w271 -> [w279]
                    tunnel: w272 -> [_]
                    # "Max Voltage"
                    # "Until it reaches 2.067"
                    # "reduce in steps of 0.5"
                    n138 = Subtract(x=w279, y=0.5) -> (x-y=w273:dbl[])
                    n139 = local write "Steps on Servo"(w273) -> ()
                    n140 = Wait (ms)(milliseconds to wait=u32 500) -> ()  [unwired: 1 out]
                    n141 = call "OnDemand_VoltageOutput.vi"("Channel Array"=w273, "minimum voltage"=0.0, "maximum voltage"=5.067, "physical channels"="cDAQ9189-21D2231Mod6/ao0") -> ()  [unwired: 7 in, 1 out]
                  }
                }
                frame #8 {
                  w280 = dbl[] [0.0]
                  # "Reset to 0"
                  # "Max Voltage"
                  n142 = call "OnDemand_VoltageOutput.vi"("Channel Array"=w280, "minimum voltage"=0.0, "maximum voltage"=5.0, "physical channels"="cDAQ9189-21D2231Mod6/ao0") -> ()  [unwired: 7 in, 1 out]
                  n143 = local write "Steps on Servo"(w280) -> ()
                }
              }
              n144 = while {
                stop <- w208 stop-if-true
                n145 = call "Elapsed Time2"() -> ("Elapsed Time (s)"=w206:dbl)  [unwired: 12 in, 7 out]
                "Elapsed Time (s) 2" <- w206
                n146 = global read "STOP_GLOBAL.vi" "ALL STOP"() -> (w208:bool)
                n147 = Greater?(x=w206, y=3.0 ("x")) -> (0:→"HAS 3 SECONDS PASSED?":bool)
              }
            }
          }
        }
        frame "Do nothing" {
        }
      }
      n148 = property on="Waveform Chart 2" class="WFChart (strict)"("History Data"=cluster{"setpoint":dbl, dbl}[] []) -> ()  [unwired: 2 in, 2 out]
      n149 = call "NI_9219_Config.vi"() -> ("error out"=w43:errorcluster, "task out"=w51:refnum<k21>)  [unwired: 10 in]
      n150 = call "NI 9237_Config.vi"("error in"=w43, "task in"=w51) -> ("error out"=w49:errorcluster, "task out"=w50:refnum<k21>)  [unwired: 8 in]
      n151 = call "NI_9210_Config.vi"("error in"=w49, "task in"=w50) -> ("error out"=w47:errorcluster, "task out"=w48:refnum<k21>)  [unwired: 8 in]
      n152 = call "NI_9252_Config.vi"("error in"=w47, "task in"=w48) -> ("error out"=w45:errorcluster, "task out"=w46:refnum<k21>)  [unwired: 8 in]
      n153 = call-poly <vilib>:"DAQmx Timing.vi"("task/channels in"=w46, "sample mode"=w58, "samples per channel"="number of samples", "rate"="rate", "active edge"=w59, "error in"=w45) -> ("task out"=w57:refnum<k21>, "error out"=w56:errorcluster)  [unwired: 8 in]
      n154 = call <vilib>:"DAQmx Start Task.vi"("task/channels in"=w57, "error in"=w56) -> ("task out"=w55:refnum<k21>, "error out"=w54:errorcluster)  [unwired: 12 in]
      n155 = while {
        tunnel: "Types of Testing" -> [w288]
        tunnel: [w334] -> w39 mode=indexing
        tunnel: w60 -> [w329]
        tunnel: "number of samples" -> [w327]
        shift-right: [w321] -> w52
        shift-left: w54 -> [w326]
        shift-right: [w293] -> w53
        shift-left: w55 -> [w325]
        tunnel: [w304] -> w40 mode=indexing
        tunnel: [w302] -> w33 mode=indexing
        tunnel: [w301] -> w41 mode=indexing
        tunnel: [w300] -> w42 mode=indexing
        tunnel: [w295] -> w24 mode=indexing
        tunnel: [w294] -> w32 mode=indexing
        tunnel: [w303] -> w31 mode=indexing
        i -> [w335]
        stop <- w330 stop-if-true
        w315 = 110.0 ("x")
        w332 = 1000.0  # timeout (s)
        # "Add SetPoint History\nAdd Gain history to data"
        # "First Test:\n2.1\n70\n3.566\nSecond:\n2.1\n80\n3.566\nThird:\n3.1\n60\n3.566\nFourth:\n10.1\n70\n3.566"
        # "Supply\nSecond Transducer\nFlow\nTemp\nOutput Voltage"
        # "4 NI 9219 Channels"
        # "Combined Loop cDAQ"
        n156 = Wait (ms)(milliseconds to wait=u32 10) -> ()  [unwired: 1 out]
        n157 = call-poly <vilib>:"DAQmx Read.vi"("task/channels in"=w325, "number of samples per channel"=w327, "timeout"=w332, "error in"=w326) -> ("task out"=w293:refnum<k21>, "data"=w328:waveform(dbl)[], "error out"=w321:errorcluster)  [unwired: 9 in]
        n158 = global read "STOP_GLOBAL.vi" "ALL STOP"() -> (w331:bool)
        n159 = Split Signals(w328) -> (w299:dynamicdata, w286:dynamicdata, w320:dynamicdata, w319:dynamicdata, w318:dynamicdata, w317:dynamicdata, w287:dynamicdata)  [unwired: 15 in, 8 out]
        n160 = Unbundle By Name(w321) -> ("status"=w333:bool)
        n161 = Or(x=w333, y=w331) -> (x .or. y?=w330:bool)
        n162 = local write "Thrust lb"(w299) -> ()
        n163 = local write "Temperature"(w286) -> ()
        n164 = Merge Signals(w320, w319, w318, w317, w287) -> (w316:dynamicdata)
        n165 = call "Filter3"("Signal"=w316) -> ("Filtered Signal"=w313:dynamicdata)  [unwired: 9 in, 1 out]
        n166 = Split Signals(w313) -> (w292:dynamicdata, w291:dynamicdata, w290:dynamicdata, w289:dynamicdata, w284:dynamicdata)  [unwired: 5 in]
        n167 = Merge Signals(w292, w291, w289, w286, w284) -> (w323:dynamicdata)
        n168 = local write "Voltage Output"(w284) -> ()
        n169 = Merge Signals(w292, w291, w290, w289, w299, w286, w284) -> (w285:dynamicdata)
        n170 = Multiply(x=w315, y=w292) -> (x*y=w312:dynamicdata)
        n171 = Multiply(x=w315, y=w291) -> (x*y=w309:dynamicdata)
        n172 = Multiply(x=w315, y=w290) -> (x*y=w308:dynamicdata)
        n173 = Multiply(x=200.0, y=w289) -> (x*y=w306:dynamicdata)
        n174 = case shown="\"Test Firing\", Default" w288 {
          tunnel: w329 -> [w349 w361]
          tunnel: w323 -> [_ w360]
          tunnel: w285 -> [w343 _]
          frame "Test Firing", Default {
            n175 = Build Array("Supply Pressure", "Second Pressure Transducer", "Chamber Pressure", "Volumetric Flow", "Thrust", "Temperature", "Voltage Out" ("element")) -> (w341:string[])
            n176 = call "RenameDynamicSignals.vi"("New Signal Names"=w341, "Dynamic Data In"=w343) -> ("error out"=w339:errorcluster, "Dynamic Data Out"=w340:dynamicdata)  [unwired: 2 in]
            n177 = call "Write To Measurement File3"("Signals"=w340, "Enable"="Collect Data?", "error in (no error)"=w339, "Filename"=w349) -> ("Filename Out"=→"Filename Out":path, "Saving Data"=→"Saving Data":bool, "error out"=→"error out 3":errorcluster)  [unwired: 13 in]
          }
          frame "Cold Flow Rig" {
            n178 = Build Array("Supply Pressure", "Second Pressure Transducer", "Volumetric Flow", "Temperature", "Voltage Out" ("element")) -> (w354:string[])
            n179 = call "RenameDynamicSignals.vi"("New Signal Names"=w354, "Dynamic Data In"=w360) -> ("error out"=w352:errorcluster, "Dynamic Data Out"=w353:dynamicdata)  [unwired: 2 in]
            n180 = call "Write To Measurement File4"("Signals"=w353, "Enable"="Collect Data? 2", "error in (no error)"=w352, "Filename"=w361) -> ("Filename Out"=→"Filename Out":path, "Saving Data"=→"Saving Data":bool)  [unwired: 13 in, 1 out]
          }
        }
        n181 = local write "Supply Pressure PSI"(w312) -> ()
        n182 = local write "Chamber Pressure"(w308) -> ()
        n183 = local write "Second Pressure Transducer"(w309) -> ()
        n184 = local write "Mass Flow L/min"(w306) -> ()
        n185 = call "Convert from Dynamic Data11"("Dynamic Data Type"=w309) -> ("Array"=w310:dbl[])  [unwired: 3 in]
        n186 = call "Convert from Dynamic Data8"("Dynamic Data Type"=w312) -> ("Array"=w311:dbl[])  [unwired: 3 in]
        n187 = call "Convert from Dynamic Data12"("Dynamic Data Type"=w308) -> ("Array"=w307:dbl[])  [unwired: 3 in]
        n188 = call "Convert from Dynamic Data13"("Dynamic Data Type"=w306) -> ("Array"=w305:dbl[])  [unwired: 3 in]
        n189 = call "Convert from Dynamic Data6"() -> ("Array"=w324:dbl[])  [unwired: 4 in]
        n190 = call-poly <vilib>:"Mean.vi"("X"=w324) -> ()  [unwired: 2 out]
        n191 = call-poly <vilib>:"Mean.vi"("X"=w311) -> ("mean"=w304:dbl)  [unwired: 1 out]
        n192 = call-poly <vilib>:"Mean.vi"("X"=w310) -> ("mean"=w303:dbl)  [unwired: 1 out]
        n193 = call-poly <vilib>:"Mean.vi"("X"=w307) -> ("mean"=w302:dbl)  [unwired: 1 out]
        n194 = call-poly <vilib>:"Mean.vi"("X"=w305) -> ("mean"=w301:dbl)  [unwired: 1 out]
        n195 = call "Convert from Dynamic Data3"("Dynamic Data Type"=w286) -> ("Array"=w297:dbl[])  [unwired: 3 in]
        n196 = call "Convert from Dynamic Data4"("Dynamic Data Type"=w284) -> ("Array"=w296:dbl[])  [unwired: 3 in]
        n197 = call "Convert from Dynamic Data"("Dynamic Data Type"=w299) -> ("Array"=w298:dbl[])  [unwired: 3 in]
        n198 = call-poly <vilib>:"Mean.vi"("X"=w296) -> ("mean"=w295:dbl)  [unwired: 1 out]
        n199 = call-poly <vilib>:"Mean.vi"("X"=w298) -> ("mean"=w334:dbl)  [unwired: 1 out]
        n200 = call-poly <vilib>:"Mean.vi"("X"=w297) -> ("mean"=w300:dbl)  [unwired: 1 out]
        n201 = call "Elapsed Time"() -> ("Elapsed Time (s)"=w294:dbl)  [unwired: 12 in, 7 out]
        "Elapsed Time (s)" <- w294
        "Numeric 2" <- w335
      }
      n202 = call <vilib>:"DAQmx Clear Task.vi"("task in"=w53, "error in"=w52) -> ("error out"=→"error out 2":errorcluster)  [unwired: 13 in]
      n203 = Bundle(w32, w31) -> (w30:cluster{dbl[], dbl[]})  [unwired: 1 in]
      "Second Pressure Transducer" <- w30
      n204 = Bundle(w32, w33) -> (w29:cluster{dbl[], dbl[]})  [unwired: 1 in]
      "Chamber Pressure" <- w29
      n205 = Bundle(w32, w40) -> (w38:cluster{dbl[], dbl[]})  [unwired: 1 in]
      "Supply Pressure" <- w38
      n206 = Bundle(w32, w41) -> (w28:cluster{dbl[], dbl[]})  [unwired: 1 in]
      "MassFlow" <- w28
      n207 = Bundle(w32, w39) -> (w27:cluster{dbl[], dbl[]})  [unwired: 1 in]
      "Thrust" <- w27
      n208 = Bundle(w32, w42) -> (w26:cluster{dbl[], dbl[]})  [unwired: 1 in]
      "Temperature" <- w26
      n209 = Bundle(w32, w24) -> (→"Servo Voltage Output":cluster{dbl[], dbl[]})  [unwired: 1 in]
      n210 = Build Array(w38, w30, w29, w28, w27, w26) -> (→"All Channel Graph":cluster{dbl[], dbl[]}[])
    }
  }
